vi "ReadScanner.vi"(8 "error in (no error)":errorcluster, 11 "Station":string) -> (0 "error out":errorcluster, 3 "DATA":string)   [LabVIEW 2020]
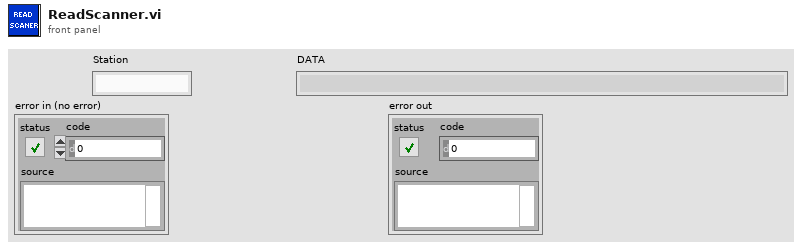
[diagram p1: front panel]
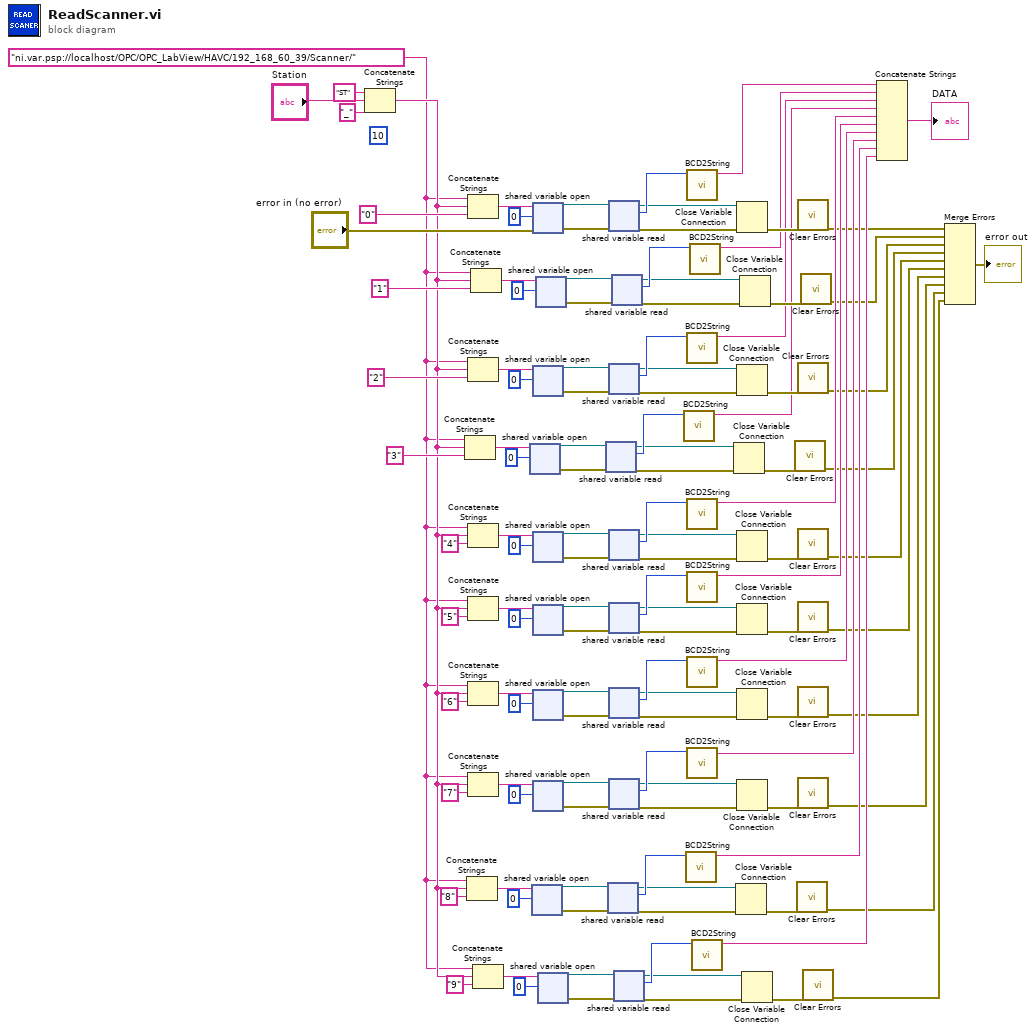
[diagram p0: block diagram]
diagram:
  (unwired) 10
  w13 = "ni.var.psp://localhost/OPC/OPC_LabView/HAVC/192_168_60_39/Scanner/"
  n1 = Concatenate Strings("ST" ("string"), "Station", "_" ("string")) -> (w14:string)
  n2 = Concatenate Strings(w13, w14, "3" ("string")) -> (w89:string)
  n3 = Concatenate Strings(w13, w14, "8" ("string")) -> (w49:string)
  n4 = Concatenate Strings(w13, w14, "0" ("string")) -> (w114:string)
  n5 = Concatenate Strings(w13, w14, "2" ("string")) -> (w97:string)
  n6 = Concatenate Strings(w13, w14, "4" ("string")) -> (w81:string)
  n7 = Concatenate Strings(w13, w14, "5" ("string")) -> (w73:string)
  n8 = Concatenate Strings(w13, w14, "6" ("string")) -> (w65:string)
  n9 = Concatenate Strings(w13, w14, "7" ("string")) -> (w57:string)
  n10 = Concatenate Strings(w13, w14, "1" ("string")) -> (w105:string)
  n11 = Concatenate Strings(w13, w14, "9" ("string")) -> (w41:string)
  n12 = shared-variable-open(w89, 0) -> (w86:refnum<k21>, w87:errorcluster)  [unwired: 2 in]
  n13 = shared-variable-open(w49, 0) -> (w46:refnum<k21>, w47:errorcluster)  [unwired: 2 in]
  n14 = shared-variable-open(w114, "error in (no error)", 0) -> (w111:refnum<k21>, w112:errorcluster)  [unwired: 1 in]
  n15 = shared-variable-open(w97, 0) -> (w94:refnum<k21>, w95:errorcluster)  [unwired: 2 in]
  n16 = shared-variable-open(w81, 0) -> (w78:refnum<k21>, w79:errorcluster)  [unwired: 2 in]
  n17 = shared-variable-open(w73, 0) -> (w70:refnum<k21>, w71:errorcluster)  [unwired: 2 in]
  n18 = shared-variable-open(w65, 0) -> (w62:refnum<k21>, w63:errorcluster)  [unwired: 2 in]
  n19 = shared-variable-open(w57, 0) -> (w54:refnum<k21>, w55:errorcluster)  [unwired: 2 in]
  n20 = shared-variable-open(w105, 0) -> (w102:refnum<k21>, w103:errorcluster)  [unwired: 2 in]
  n21 = shared-variable-open(w41, 0) -> (w38:refnum<k21>, w39:errorcluster)  [unwired: 2 in]
  n22 = shared-variable-read(w86, w87) -> (w83:refnum<k21>, w84:errorcluster, w85:i32)  [unwired: 1 out]
  n23 = shared-variable-read(w46, w47) -> (w43:refnum<k21>, w44:errorcluster, w45:i32)  [unwired: 1 out]
  n24 = shared-variable-read(w111, w112) -> (w108:refnum<k21>, w109:errorcluster, w110:i32)  [unwired: 1 out]
  n25 = shared-variable-read(w94, w95) -> (w91:refnum<k21>, w92:errorcluster, w93:i32)  [unwired: 1 out]
  n26 = shared-variable-read(w78, w79) -> (w75:refnum<k21>, w76:errorcluster, w77:i32)  [unwired: 1 out]
  n27 = shared-variable-read(w70, w71) -> (w67:refnum<k21>, w68:errorcluster, w69:i32)  [unwired: 1 out]
  n28 = shared-variable-read(w62, w63) -> (w59:refnum<k21>, w60:errorcluster, w61:i32)  [unwired: 1 out]
  n29 = shared-variable-read(w54, w55) -> (w51:refnum<k21>, w52:errorcluster, w53:i32)  [unwired: 1 out]
  n30 = shared-variable-read(w102, w103) -> (w99:refnum<k21>, w100:errorcluster, w101:i32)  [unwired: 1 out]
  n31 = shared-variable-read(w38, w39) -> (w35:refnum<k21>, w36:errorcluster, w37:i32)  [unwired: 1 out]
  n32 = call "BCD2String.vi"("BCD Int"=w85) -> ("String"=w27:string)  [unwired: 10 in]
  n33 = call "BCD2String.vi"("BCD Int"=w45) -> ("String"=w22:string)  [unwired: 10 in]
  n34 = call "BCD2String.vi"("BCD Int"=w110) -> ("String"=w30:string)  [unwired: 10 in]
  n35 = call "BCD2String.vi"("BCD Int"=w93) -> ("String"=w28:string)  [unwired: 10 in]
  n36 = call "BCD2String.vi"("BCD Int"=w77) -> ("String"=w26:string)  [unwired: 10 in]
  n37 = call "BCD2String.vi"("BCD Int"=w69) -> ("String"=w25:string)  [unwired: 10 in]
  n38 = call "BCD2String.vi"("BCD Int"=w61) -> ("String"=w24:string)  [unwired: 10 in]
  n39 = call "BCD2String.vi"("BCD Int"=w53) -> ("String"=w23:string)  [unwired: 10 in]
  n40 = call "BCD2String.vi"("BCD Int"=w101) -> ("String"=w29:string)  [unwired: 10 in]
  n41 = call "BCD2String.vi"("BCD Int"=w37) -> ("String"=w21:string)  [unwired: 10 in]
  n42 = Close Variable Connection(8:w84, 11:w83) -> (0:w82:errorcluster)
  n43 = Close Variable Connection(8:w44, 11:w43) -> (0:w42:errorcluster)
  n44 = Close Variable Connection(8:w109, 11:w108) -> (0:w107:errorcluster)
  n45 = Close Variable Connection(8:w92, 11:w91) -> (0:w90:errorcluster)
  n46 = Close Variable Connection(8:w76, 11:w75) -> (0:w74:errorcluster)
  n47 = Close Variable Connection(8:w68, 11:w67) -> (0:w66:errorcluster)
  n48 = Close Variable Connection(8:w60, 11:w59) -> (0:w58:errorcluster)
  n49 = Close Variable Connection(8:w52, 11:w51) -> (0:w50:errorcluster)
  n50 = Close Variable Connection(8:w100, 11:w99) -> (0:w98:errorcluster)
  n51 = Close Variable Connection(8:w36, 11:w35) -> (0:w34:errorcluster)
  n52 = call <vilib>:"Clear Errors.vi"("error in (no error)"=w82) -> ("error out"=w8:errorcluster)  [unwired: 5 in, 1 out]
  n53 = call <vilib>:"Clear Errors.vi"("error in (no error)"=w42) -> ("error out"=w3:errorcluster)  [unwired: 5 in, 1 out]
  n54 = call <vilib>:"Clear Errors.vi"("error in (no error)"=w107) -> ("error out"=w11:errorcluster)  [unwired: 5 in, 1 out]
  n55 = call <vilib>:"Clear Errors.vi"("error in (no error)"=w90) -> ("error out"=w9:errorcluster)  [unwired: 5 in, 1 out]
  n56 = call <vilib>:"Clear Errors.vi"("error in (no error)"=w74) -> ("error out"=w7:errorcluster)  [unwired: 5 in, 1 out]
  n57 = call <vilib>:"Clear Errors.vi"("error in (no error)"=w66) -> ("error out"=w6:errorcluster)  [unwired: 5 in, 1 out]
  n58 = call <vilib>:"Clear Errors.vi"("error in (no error)"=w58) -> ("error out"=w5:errorcluster)  [unwired: 5 in, 1 out]
  n59 = call <vilib>:"Clear Errors.vi"("error in (no error)"=w50) -> ("error out"=w4:errorcluster)  [unwired: 5 in, 1 out]
  n60 = call <vilib>:"Clear Errors.vi"("error in (no error)"=w98) -> ("error out"=w10:errorcluster)  [unwired: 5 in, 1 out]
  n61 = call <vilib>:"Clear Errors.vi"("error in (no error)"=w34) -> ("error out"=w2:errorcluster)  [unwired: 5 in, 1 out]
  n62 = Concatenate Strings(w30, w29, w28, w27, w26, w25, w24, w23, w22, w21) -> (→"DATA":string)
  n63 = Merge Errors(w11, w10, w9, w8, w7, w6, w5, w4, w3, w2) -> (→"error out":errorcluster)
